vi "Initialize Device.vi"(8 "error in (no error)":errorcluster, 9 "Number of Axes":i32, 10 "VISA resource name":refnum<visa-resource-name>, 11 "ESP301 in":refnum<class "ESP301.lvclass">) -> (0 "error out":errorcluster, 3 "ESP301 out":refnum<class "ESP301.lvclass">)   [LabVIEW 2019, in "ESP301.lvclass"]
uses:
  ESP301.lvclass
  ESP301.lvclass/ESP301.ctl
  ESP301-Driver/ESP301-Driver.lvlib
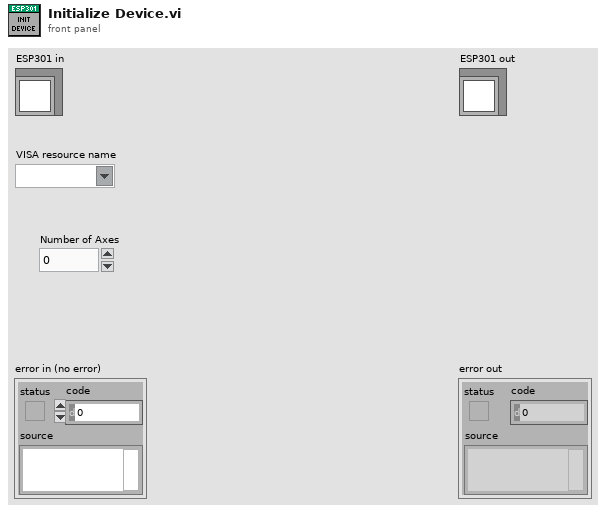
[diagram p1: front panel]
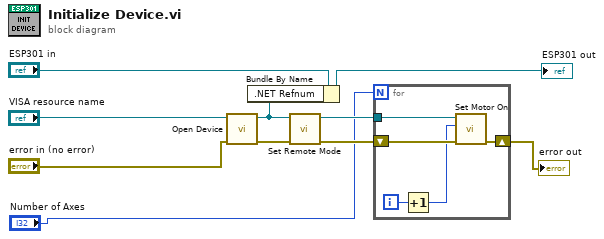
[diagram p0: block diagram]
diagram:
  n1 = call "Open Device.vi"("error in"="error in (no error)", "Port"="VISA resource name") -> ("error out"=w6:errorcluster, ".NET Refnum out"=w4:refnum<k24>)  [unwired: 8 in]
  n2 = Bundle By Name(cluster="ESP301 in", ".NET Refnum"=w4) -> (→"ESP301 out":refnum<class "ESP301.lvclass">)
  n3 = call "Set Remote Mode.vi"("error in (no error)"=w6, ".NET Refnum in"=w4) -> ("error out"=w5:errorcluster, ".NET Refnum out"=w2:refnum<k24>)  [unwired: 8 in]
  n4 = for {
    N: "Number of Axes" -> [_]
    tunnel: w2 -> [w13]
    shift-right: [w14] -> w3
    shift-left: w5 -> [w15]
    i -> [w12]
    n5 = Increment(x=w12) -> (x+1=w11:i32)
    n6 = call "Set Motor On.vi"("error in"=w15, "axisNumber"=w11, "reference"=w13) -> ("error out"=w14:errorcluster)  [unwired: 7 in, 1 out]
  }
  "error out" <- w3
